vi "P controller.vi"(7 "range":cluster{"max":dbl, "min":dbl}={"max"=100.0, "min"=-100.0}, 8 "dt (s)":dbl, 9 "P gain":dbl, 10 "process variable":dbl, 11 "setpoint":dbl) -> (0 "dt (s)":dbl, 2 "output":dbl)   [LabVIEW 2009]
doc: "This VI is a faster control loop than PID when only the P term is needed."
panel:
  # "P  I  D"
  # "http://en.wikipedia.org/wiki/PID_controller"
  # "This VI is compatible with the LabVIEW NXT toolkit 2.0"
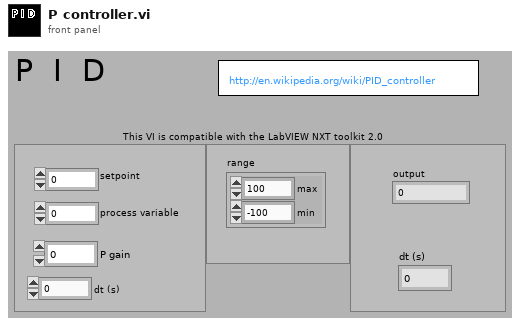
[diagram p1: front panel]
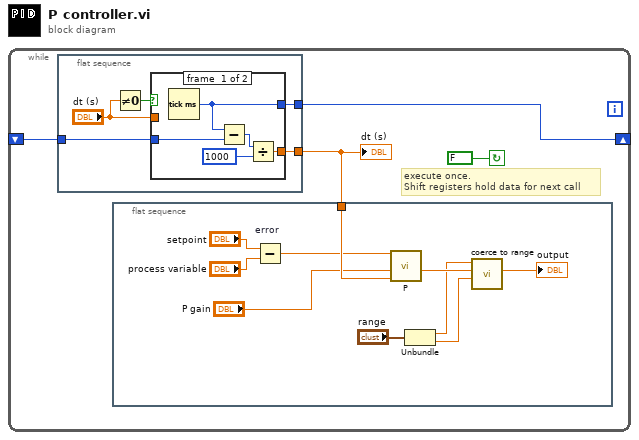
[diagram p0: block diagram]
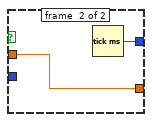
[diagram p2: hidden frame]
diagram:
  n1 = while {
    shift-right: [w2] -> _
    shift-left: _ -> [w3]
    stop <- FALSE continue-if-true
    # "execute once.\nShift registers hold data for next call"
    n2 = flat-sequence {
      tunnel: w3 -> [w19]
      tunnel: [w18] -> w2
      tunnel: [w17] -> w1
      frame #0 {
        n3 = Not Equal To 0?(x="dt (s)") -> (x != 0?=w16:bool)
        n4 = case shown="True" w16 {
          tunnel: w19 -> [w24 _]
          tunnel: [w23 w25] -> w18
          tunnel: [w20 w26] -> w17
          tunnel: "dt (s)" -> [_ w26]
          frame #0 {
            n5 = Tick Count (ms)() -> (millisecond timer value=w23:u32)
            n6 = Subtract(x=w23, y=w24) -> (x-y=w22:u32)
            n7 = Divide(x=w22, y=u32 1000) -> (x/y=w20:dbl)
          }
          frame #1 {
            n8 = Tick Count (ms)() -> (millisecond timer value=w25:u32)
          }
        }
      }
    }
    n9 = flat-sequence {
      tunnel: w1 -> [w14]
      frame #0 {
        n10 = Subtract "error"(x="setpoint", y="process variable") -> (x-y=w11:dbl)
        n11 = call "P.vi"("change time"=w14, "P gain"="P gain", "error"=w11) -> ("output"=w9:dbl)  [unwired: 8 in]
        n12 = Unbundle("range") -> ("max"=w6:dbl, "min"=w7:dbl)
        n13 = call "coerce to range.vi"("min"=w7, "value in"=w9, "max"=w6) -> ("value out"=→"output":dbl)  [unwired: 7 in, 1 out]
      }
    }
    "dt (s)" <- w1
  }
